vi "FTW-Example-SlasdClient-Core-Process.vi"() -> ()   [LabVIEW 2013, in "FTW-Example-SlasdClient-Core.lvclass"]
uses:
  FTW-Example-SlasdClient-Core.lvclass
  source/actor/Message/Base/FTW-Message.lvclass
  FTW-Example-SlasdClient-Core.lvclass/FTW-Example-SlasdClient-Core.ctl
  SLASD/FTW-Example-SLASD.lvclass
  source/actor/Instance/FTW-ActorInstance.lvclass/FTW-ActorInstance.ctl
  source/actor/JobSequencer/FTW-SEQ-Current.vi
  source/actor/Instance/FTW-ActorInstance.lvclass
  source/actor/Message/Request/FTW-Message-IncomingRequest.lvclass
  source/actor/Ether/FTW-Ether.lvclass
  source/actor/Connector/FTW-ActorConnector.lvclass
panel:
  out "Roundtrip Time":dbl
  in  "Timeout":i32=1000 format="%dmsec"
  in  "Request Body":string
  in  "Request Header":string
  in  "Send Message to SLASD":bool
  out "Response Header":string
  out "Response Body":string
  out "Timed out?":bool
  out "PoisonPill Timed out?":bool
  out "PoisonPill Response Body":string
  out "PoisonPill Response Header":string
  in  "Shutdown SLASD":bool
  out "Heartbeat":bool
  out "SLASD Status":string
  in  "SLASD IP Address":string(combo)
  # "send the shutdown message"
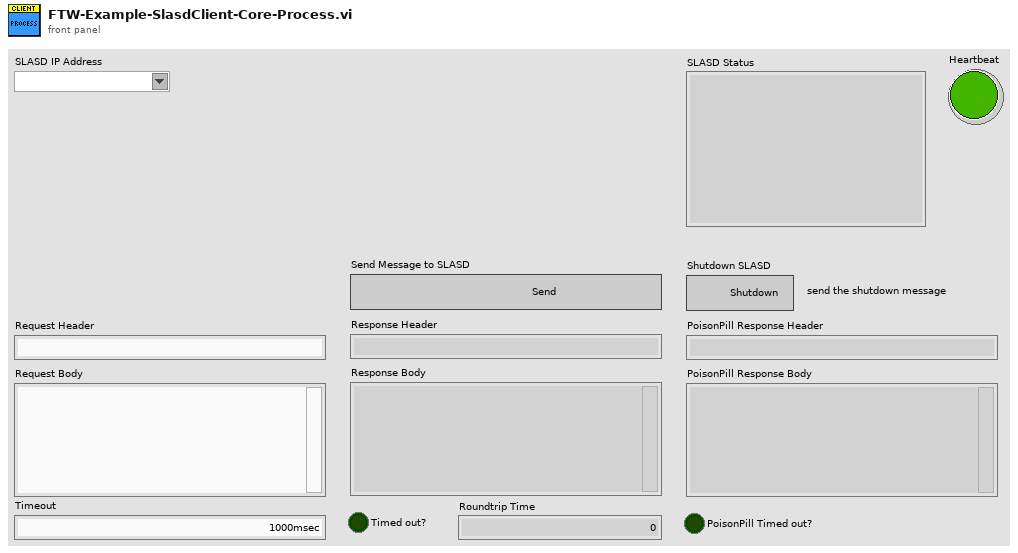
[diagram p1: front panel]
types:
  T1 = cluster{"Incoming Requests":refnum<event-registration>, "SLASD Subscription":refnum<event-registration>}
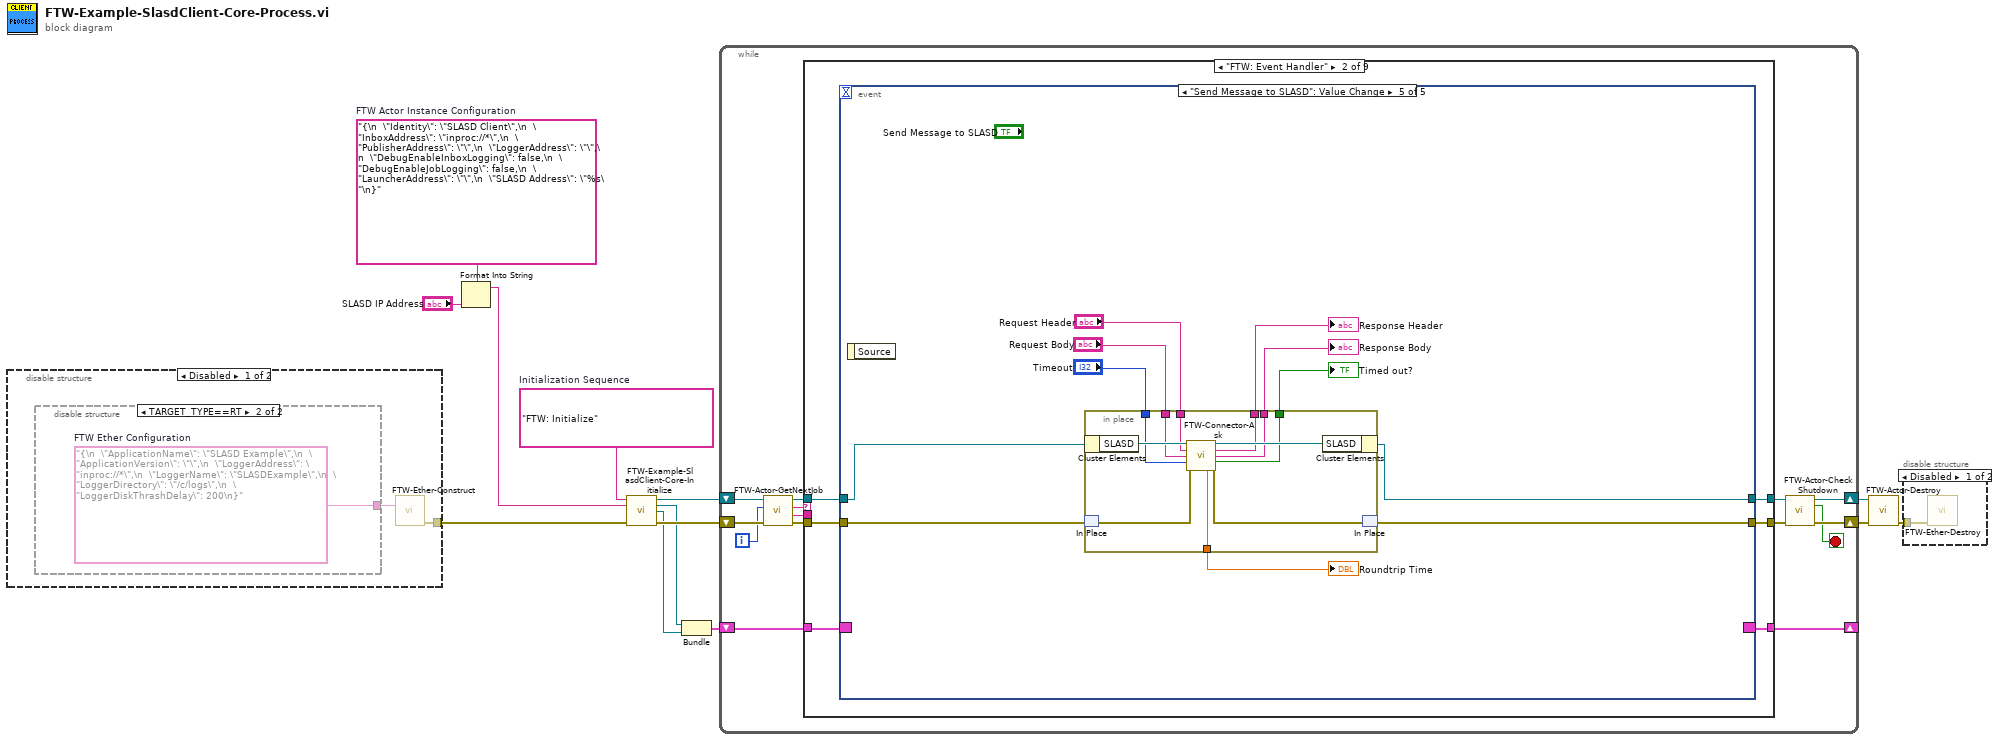
[diagram p0: block diagram]
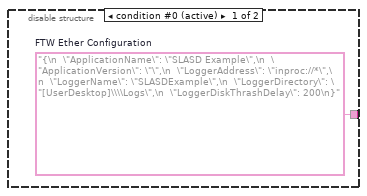
[diagram p3: hidden frame]
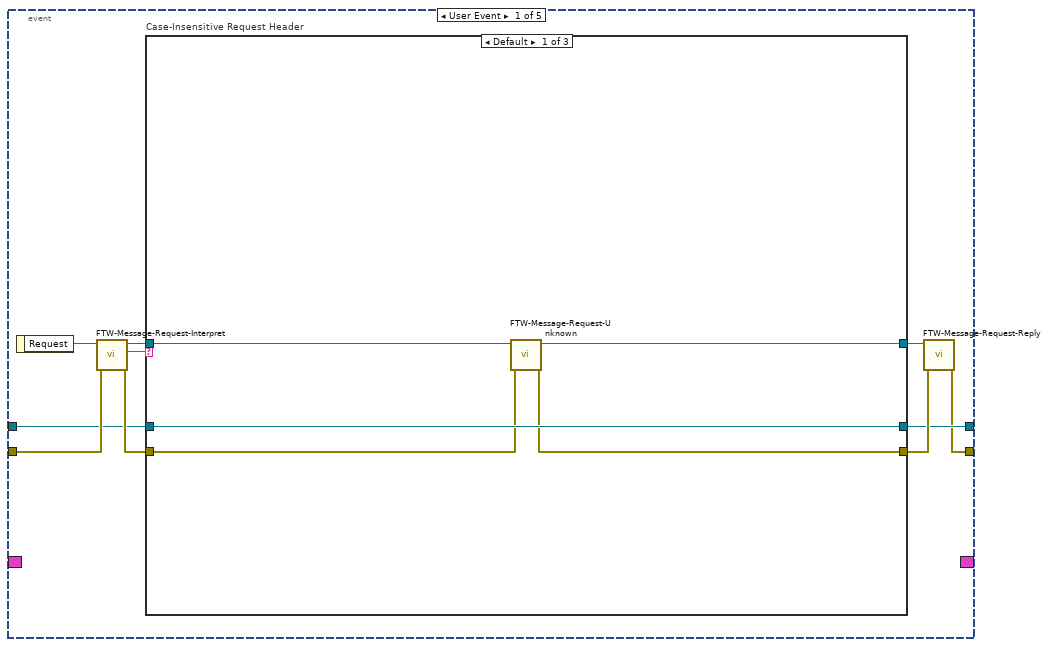
[diagram p6: hidden frame]
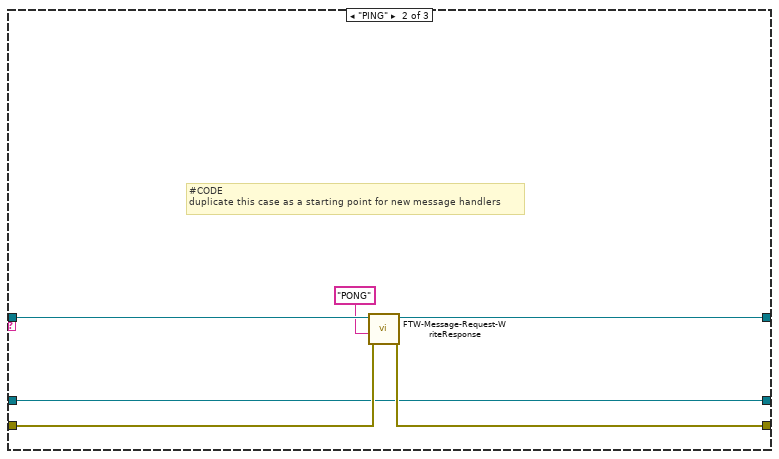
[diagram p7: hidden frame]
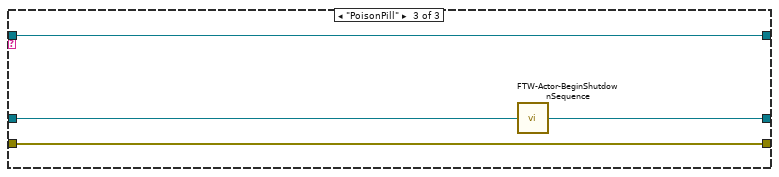
[diagram p8: hidden frame]
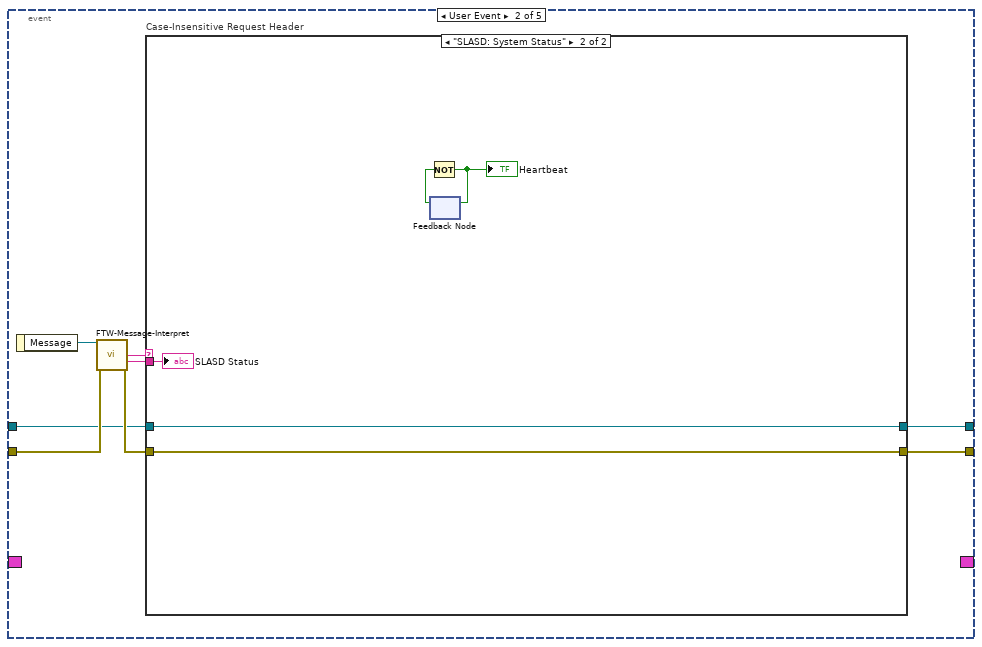
[diagram p9: hidden frame]
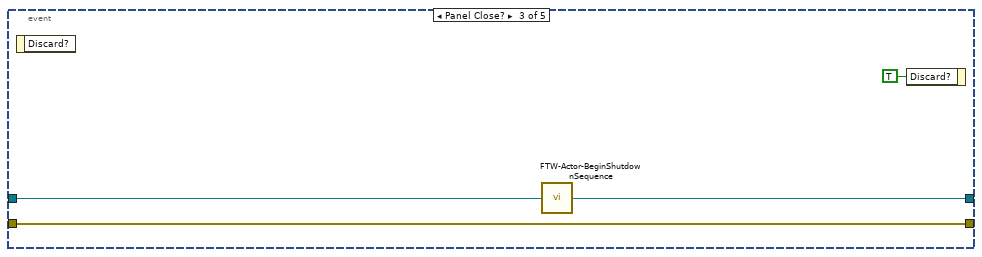
[diagram p11: hidden frame]
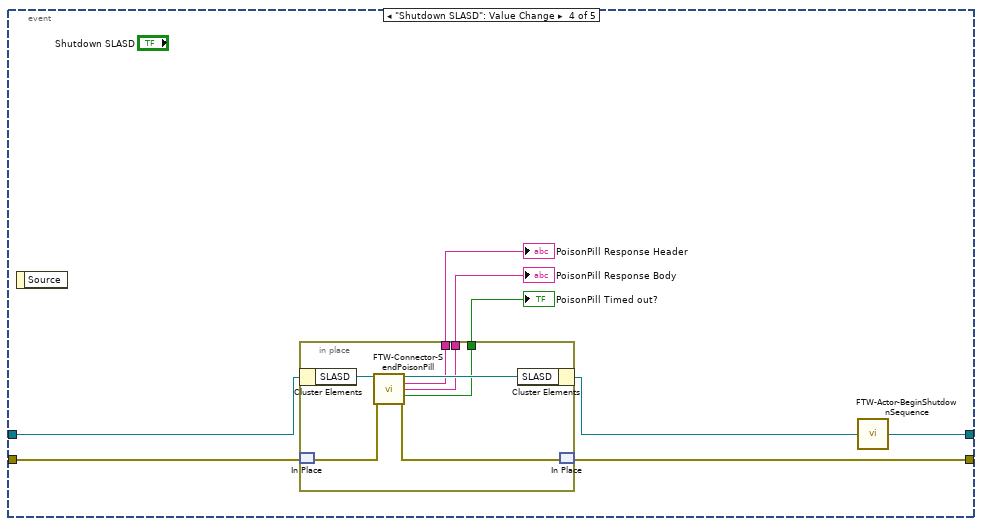
[diagram p12: hidden frame]
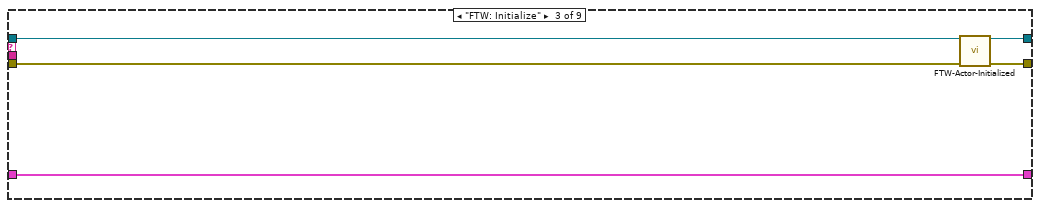
[diagram p13: hidden frame]
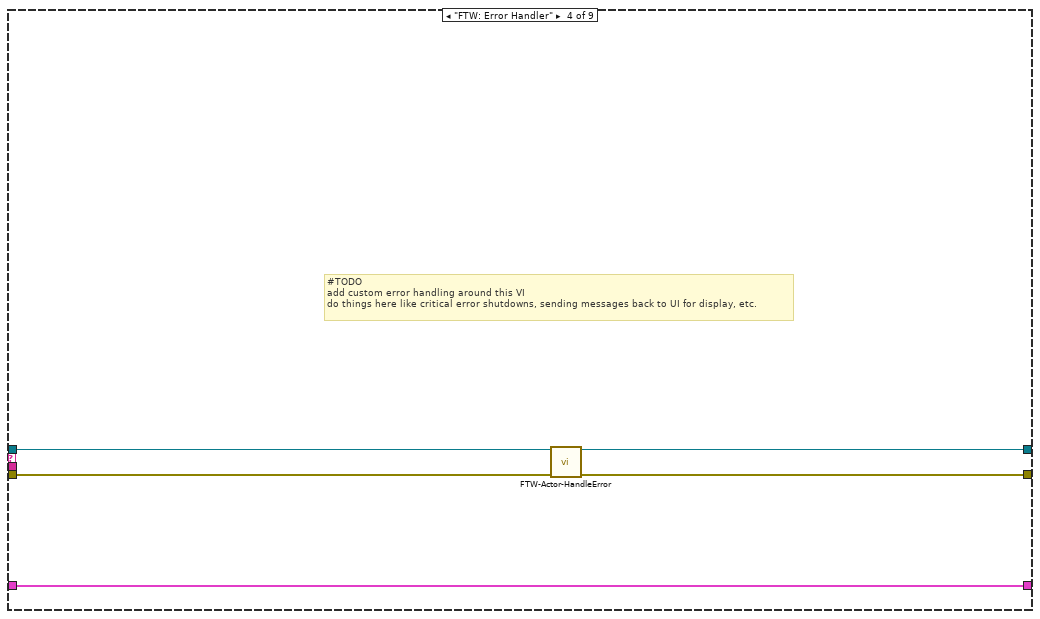
[diagram p14: hidden frame]
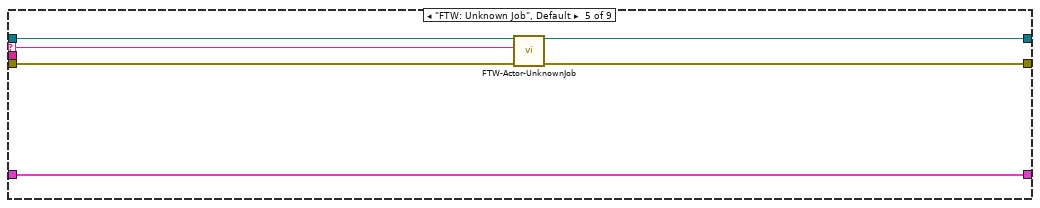
[diagram p15: hidden frame]
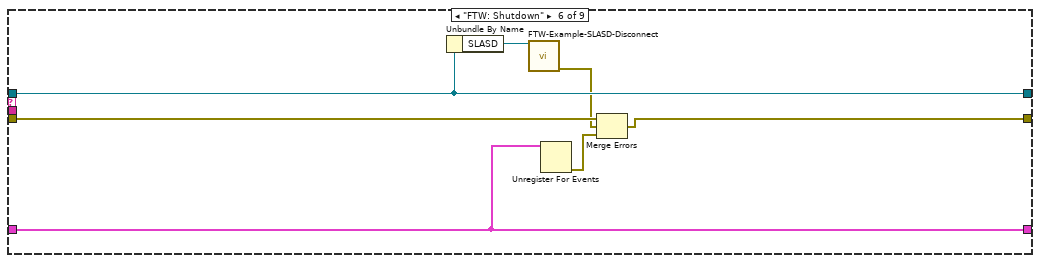
[diagram p16: hidden frame]
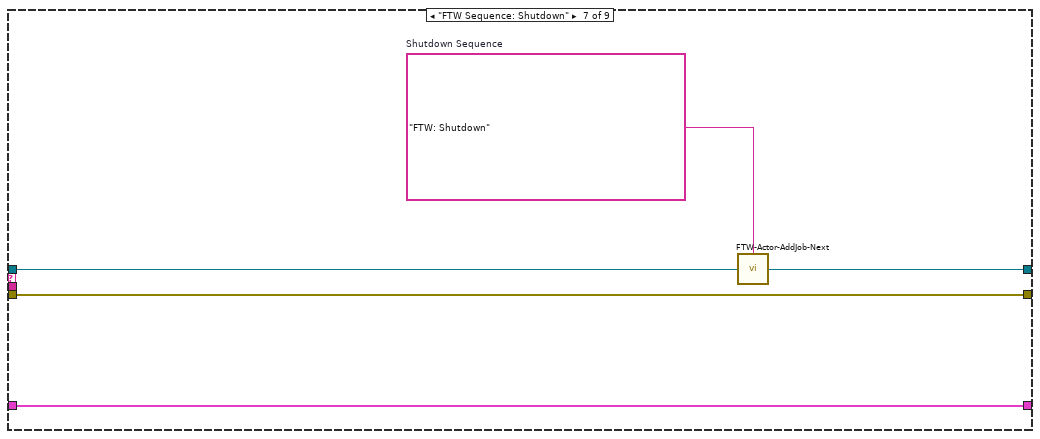
[diagram p17: hidden frame]
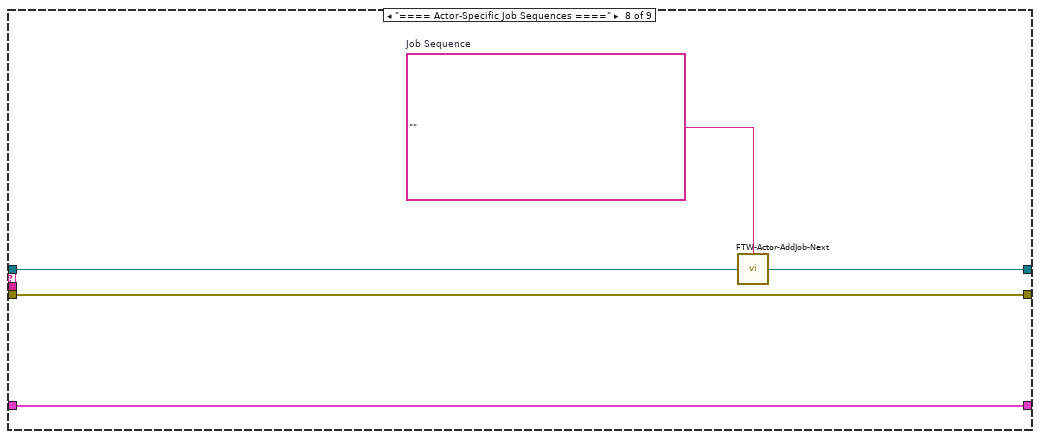
[diagram p18: hidden frame]
diagram:
  w3 = "{\n  \"Identity\": \"SLASD Client\",\n  \"InboxAddress\": \"inproc://*\",\n  \"PublisherAddress\": \"\",\n  \"LoggerAddress\": \"\",\n  \"DebugEnableInboxLogging\": false,\n  \"DebugEnableJobLogging\": false,\n  \"LauncherAddress\": \"\",\n  \"SLASD Address\": \"%s\"\n}"  # FTW Actor Instance Configuration
  w8 = "FTW: Initialize"  # Initialization Sequence
  n1 = disable-structure shown="Disabled" {
    disable-tunnel: [w15 _] -> w5
    frame Disabled {
      n2 = disable-structure shown="TARGET_TYPE==RT" {
        disable-tunnel: [w16 w17] -> w14
        frame condition #0 (active) {
          w16 = "{\n  \"ApplicationName\": \"SLASD Example\",\n  \"ApplicationVersion\": \"\",\n  \"LoggerAddress\": \"inproc://*\",\n  \"LoggerName\": \"SLASDExample\",\n  \"LoggerDirectory\": \"[UserDesktop]\\\\Logs\",\n  \"LoggerDiskThrashDelay\": 200\n}"  # FTW Ether Configuration
        }
        frame condition #1 {
          w17 = "{\n  \"ApplicationName\": \"SLASD Example\",\n  \"ApplicationVersion\": \"\",\n  \"LoggerAddress\": \"inproc://*\",\n  \"LoggerName\": \"SLASDExample\",\n  \"LoggerDirectory\": \"/c/logs\",\n  \"LoggerDiskThrashDelay\": 200\n}"  # FTW Ether Configuration
        }
      }
      n3 = call "FTW-Ether-Construct.vi"("FTW Ether Configuration"=w14) -> ("error out"=w15:errorcluster)  [unwired: 14 in]
    }
    frame Enabled {
    }
  }
  n4 = Format Into String(format string=w3, "SLASD IP Address") -> (resulting string=w2:string)  [unwired: 2 in, 1 out]
  n5 = call "FTW-Example-SlasdClient-Core-Initialize.vi"("Initialization Sequence"=w8, "FTW Actor Instance Configuration"=w2, "error in (no error)"=w5) -> ("Actor Template-Core out"=w13:refnum<class "FTW-Example-SlasdClient-Core.lvclass">, "Incoming Requests"=w6:refnum<event-registration>, "SLASD Subscription"=w4:refnum<event-registration>, "error out"=w9:errorcluster)  [unwired: 9 in]
  n6 = Bundle("Incoming Requests"=w6, "SLASD Subscription"=w4) -> (w7:T1)  [unwired: 1 in]
  n7 = while {
    shift-right: [w21] -> w11
    shift-left: w9 -> [w28]
    shift-right: [w18] -> _
    shift-left: w7 -> [w31]
    shift-right: [w23] -> w12
    shift-left: w13 -> [w30]
    i -> [w19]
    stop <- w20 stop-if-true
    n8 = call "FTW-Actor-GetNextJob.vi"("error in"=w28, "Jobs Performed"=w19, "FTW Actor Instance"=w30) -> ("error out"=w27:errorcluster, "Job Data"=w25:string, "Job Name"=w26:string, "FTW Actor Instance out"=w29:refnum<class "FTW-Example-SlasdClient-Core.lvclass">)  [unwired: 5 in]
    n9 = case shown="\"FTW: Event Handler\"" w26 {
      selector: w26 -> [_ _ _ _ w132 _ _ _ _]
      tunnel: [w33 w40 w122 w127 w135 w143 w148 w153 w157] -> w22
      tunnel: w27 -> [w33 w39 w125 w129 w136 w144 w148 w153 w157]
      tunnel: w31 -> [w34 w35 w126 w131 w137 w141 w149 w154 w156]
      tunnel: [w34 w38 w126 w131 w137 w141 w149 w154 w156] -> w18
      tunnel: w25 -> [_ _ _ _ _ _ _ _ _]
      tunnel: [w32 w37 w123 w128 w133 w140 w146 w151 w155] -> w24
      tunnel: w29 -> [w32 w36 w124 w130 w134 w140 w147 w152 w155]
      frame "==== Featherweight Framework Jobs ====" {
      }
      frame "FTW: Event Handler" {
        n10 = event shown="[4] \"Send Message to SLASD\": Value Change" {
          selector: w35 -> [_ _ _ _ _]
          dyn-events: [_ _ _ _ _] -> w38
          timeout: _ -> [_ _ _ _ _]
          tunnel: [w43 w72 w83 w88 w107] -> w40
          tunnel: w39 -> [w42 w69 w83 w89 w108]
          tunnel: [w44 w70 w81 w92 w109] -> w37
          tunnel: w36 -> [w41 w68 w82 w91 w110]
          event User Event {
            n11 = event-data() -> ("Request"=w45:refnum<class "FTW-Message-IncomingRequest.lvclass">)  [unwired: 1 in]
            n12 = call "FTW-Message-Request-Interpret.vi"("error in"=w42, "FTW Incoming Request"=w45) -> ("error out"=w50:errorcluster, "Request Header"=w48:string, "FTW Incoming Request out"=w47:refnum<class "FTW-Message-IncomingRequest.lvclass">)  [unwired: 5 in, 2 out]
            n13 = case "Case-Insensitive Request Header" shown="Default" w48 {
              tunnel: [w53 w59 w64] -> w49
              tunnel: w50 -> [w54 w60 w64]
              tunnel: [w55 w58 w65] -> w44
              tunnel: w41 -> [w55 w58 w63]
              tunnel: w47 -> [w52 w61 w62]
              tunnel: [w51 w57 w62] -> w46
              frame Default {
                n14 = call "FTW-Message-Request-Unknown.vi"("error in"=w54, "FTW Incoming Request"=w52) -> ("error out"=w53:errorcluster, "FTW Incoming Request Out"=w51:refnum<class "FTW-Message-IncomingRequest.lvclass">)  [unwired: 8 in]
              }
              frame "PING" {
                # "#CODE\nduplicate this case as a starting point for new message handlers"
                n15 = call "FTW-Message-Request-WriteResponse.vi"("error in"=w60, "Response Body"="PONG" ("Response Header"), "FTW Incoming Request"=w61) -> ("error out"=w59:errorcluster, "FTW Incoming Request out"=w57:refnum<class "FTW-Message-IncomingRequest.lvclass">)  [unwired: 7 in]
              }
              frame "PoisonPill" {
                n16 = call "FTW-Actor-BeginShutdownSequence.vi"("FTW Actor Instance"=w63) -> ("FTW Actor Instance out"=w65:refnum<class "FTW-Example-SlasdClient-Core.lvclass">)  [unwired: 3 in]
              }
            }
            n17 = call "FTW-Message-Request-Reply.vi"("FTW: Reply Error"=w49, "FTW Incoming Request"=w46) -> ("error out"=w43:errorcluster)  [unwired: 8 in, 1 out]
          }
          event User Event {
            n18 = event-data() -> ("Message"=w71:refnum<class "FTW-Message.lvclass">)  [unwired: 1 in]
            n19 = call-dynamic "FTW-Message-Interpret.vi"("FTW Message"=w71, "error in"=w69) -> ("Message Header"=w67:string, "Message Body"=w66:string, "error out"=w73:errorcluster)  [unwired: 9 in, 2 out]
            n20 = case "Case-Insensitive Request Header" shown="\"SLASD: System Status\"" w67 {
              tunnel: [w74 w79] -> w72
              tunnel: w73 -> [w74 w79]
              tunnel: [w75 w80] -> w70
              tunnel: w68 -> [w75 w80]
              tunnel: w66 -> [_ w78]
              frame Default {
              }
              frame "SLASD: System Status" {
                n21 = feedback #1() -> (w77:bool)  [unwired: 1 in]
                n22 = Not(x=w77) -> (.not. x?=w76:bool)
                "Heartbeat" <- w76
                n23 = feedback-in #1(w76) -> ()
                "SLASD Status" <- w78
              }
            }
          }
          event Panel Close? {
            n24 = event-data() -> ()  [unwired: 1 in, 1 out]
            n25 = call "FTW-Actor-BeginShutdownSequence.vi"("FTW Actor Instance"=w82) -> ("FTW Actor Instance out"=w81:refnum<class "FTW-Example-SlasdClient-Core.lvclass">)  [unwired: 3 in]
            n26 = event-data("Discard?"=TRUE) -> ()  [unwired: 1 in, 1 out]
          }
          event "Shutdown SLASD": Value Change {
            n27 = event-data() -> ()  [unwired: 1 in, 1 out]
            n28 = in-place {
              in-place-border: [w95] -> w87
              in-place-border: [w94] -> w86
              in-place-border: [w93] -> w85
              n29 = in-place-cluster #2(w91) -> ("SLASD"=w97:refnum<class "FTW-Example-SLASD.lvclass">)
              n30 = in-place-match #3(w89) -> (w99:errorcluster)
              n31 = call-dynamic "FTW-Connector-SendPoisonPill.vi"("FTW Actor Connector"=w97, "error in"=w99) -> ("FTW Actor Connector out"=w96:refnum<class "FTW-Example-SLASD.lvclass">, "Response Header"=w95:string, "Response Body"=w94:string, "Timed out?"=w93:bool, "error out"=w98:errorcluster)  [unwired: 9 in]
              n32 = in-place-cluster #2("SLASD"=w96) -> (w90:refnum<class "FTW-Example-SlasdClient-Core.lvclass">)
              n33 = in-place-match #3(w98) -> (w88:errorcluster)
            }
            "PoisonPill Response Header" <- w87
            "PoisonPill Response Body" <- w86
            "PoisonPill Timed out?" <- w85
            n34 = call "FTW-Actor-BeginShutdownSequence.vi"("FTW Actor Instance"=w90) -> ("FTW Actor Instance out"=w92:refnum<class "FTW-Example-SlasdClient-Core.lvclass">)  [unwired: 3 in]
          }
          event "Send Message to SLASD": Value Change {
            n35 = event-data() -> ()  [unwired: 1 in, 1 out]
            n36 = in-place {
              in-place-border: [w117] -> w106
              in-place-border: [w116] -> w105
              in-place-border: [w115] -> w104
              in-place-border: "Request Header" -> [w114]
              in-place-border: "Request Body" -> [w113]
              in-place-border: "Timeout" -> [w112]
              in-place-border: [w111] -> w100
              n37 = in-place-cluster #4(w110) -> ("SLASD"=w119:refnum<class "FTW-Example-SLASD.lvclass">)
              n38 = in-place-match #5(w108) -> (w121:errorcluster)
              n39 = call "FTW-Connector-Ask.vi"("FTW Actor Connector"=w119, "Request Header"=w114, "Request Body"=w113, "Timeout"=w112, "error in"=w121) -> ("FTW Actor Connector out"=w118:refnum<class "FTW-Example-SLASD.lvclass">, "Response Header"=w117:string, "Response Body"=w116:string, "Timed out?"=w115:bool, "Roundtrip Time"=w111:dbl, "error out"=w120:errorcluster)  [unwired: 4 in, 1 out]
              n40 = in-place-cluster #4("SLASD"=w118) -> (w109:refnum<class "FTW-Example-SlasdClient-Core.lvclass">)
              n41 = in-place-match #5(w120) -> (w107:errorcluster)
            }
            "Response Header" <- w106
            "Response Body" <- w105
            "Timed out?" <- w104
            "Roundtrip Time" <- w100
          }
        }
      }
      frame "FTW: Initialize" {
        n42 = call-dynamic "FTW-Actor-Initialized.vi"("FTW Actor Instance"=w124, "error in"=w125) -> ("FTW Actor Instance out"=w123:refnum<class "FTW-Example-SlasdClient-Core.lvclass">, "error out"=w122:errorcluster)  [unwired: 12 in]
      }
      frame "FTW: Error Handler" {
        # "#TODO\nadd custom error handling around this VI\ndo things here like critical error shutdowns, sending messages back to UI for display, etc."
        n43 = call-dynamic "FTW-Actor-HandleError.vi"("FTW Actor Instance"=w130, "error in"=w129) -> ("FTW Actor Instance out"=w128:refnum<class "FTW-Example-SlasdClient-Core.lvclass">, "error out"=w127:errorcluster)  [unwired: 10 in, 2 out]
      }
      frame "FTW: Unknown Job", Default {
        n44 = call-dynamic "FTW-Actor-UnknownJob.vi"("FTW Actor Instance"=w134, "Unknown Job"=w132, "error in"=w136) -> ("FTW Actor Instance out"=w133:refnum<class "FTW-Example-SlasdClient-Core.lvclass">, "error out"=w135:errorcluster)  [unwired: 11 in]
      }
      frame "FTW: Shutdown" {
        n45 = Unbundle By Name(w140) -> ("SLASD"=w139:refnum<class "FTW-Example-SLASD.lvclass">)
        n46 = call "FTW-Example-SLASD-Disconnect.vi"("FTW-Example-SLASD In"=w139) -> ("error out"=w138:errorcluster)  [unwired: 14 in]
        n47 = Unregister For Events(event registration refnum=w141) -> (error out=w142:errorcluster)  [unwired: 1 in]
        n48 = Merge Errors(w144, w138, w142) -> (w143:errorcluster)
      }
      frame "FTW Sequence: Shutdown" {
        w145 = "FTW: Shutdown"  # Shutdown Sequence
        n49 = call "FTW-Actor-AddJob-Next.vi"("Add Next in Job Queue"=w145, "FTW Actor Instance"=w147) -> ("FTW Actor Instance out"=w146:refnum<class "FTW-Example-SlasdClient-Core.lvclass">)  [unwired: 2 in]
      }
      frame "==== Actor-Specific Job Sequences ====" {
        w150 = ""  # Job Sequence
        n50 = call "FTW-Actor-AddJob-Next.vi"("Add Next in Job Queue"=w150, "FTW Actor Instance"=w152) -> ("FTW Actor Instance out"=w151:refnum<class "FTW-Example-SlasdClient-Core.lvclass">)  [unwired: 2 in]
      }
      frame "==== Actor-Specific Jobs ====" {
      }
    }
    n51 = call "FTW-Actor-CheckShutdown.vi"("FTW Actor Instance"=w24, "error in"=w22) -> ("FTW Actor Instance out"=w23:refnum<class "FTW-Example-SlasdClient-Core.lvclass">, "Shutdown?"=w20:bool, "error out"=w21:errorcluster)  [unwired: 11 in]
  }
  n52 = call-dynamic "FTW-Actor-Destroy.vi"("FTW Actor Instance"=w12, "error in"=w11) -> ("error out"=w10:errorcluster)  [unwired: 13 in]
  n53 = disable-structure shown="Disabled" {
    disable-tunnel: w10 -> [w158 _]
    frame Disabled {
      n54 = call "FTW-Ether-Destroy.vi"("error in"=w158) -> ()  [unwired: 14 in, 1 out]
    }
    frame Enabled {
    }
  }
